vi "FORTESTING.vi"   [LabVIEW 2016, in "Test2.lvrbt"]
uses:
  Test2.lvrbt
  <vilib>/NXT/Subs/ColorSensorColors.ctl
  <vilib>/NXT/Block Support/NXT_InputPort.ctl
  <vilib>/NXT/Hardware/Plugins/Tetrix DC Motor/TetrixDCMotorAddress.ctl
  <vilib>/NXT/Hardware/Plugins/Tetrix 180 deg Servo/Tetrix180ServoAddress.ctl
  <vilib>/NXT/NXTIO Xnodes/NXTIONodeSubVIs/TETRIX IO Move DC Motors.vi
  <vilib>/NXT/Dual Mode Library/Waits/Wait_Num.vi
  <vilib>/NXT/NXTIO Xnodes/NXTIONodeSubVIs/TETRIX IO Stop DC Motors.vi
  <vilib>/NXT/Dual Mode Library/Waits/Wait_EV3_Color_Color.vi
  <vilib>/NXT/NXTIO Xnodes/NXTIONodeSubVIs/TETRIX IO Move Servos.vi
  <vilib>/NXT/Dual Mode Library/Waits/Wait_EV3_Ultrasonic_Centimeter_Closer.vi
  <vilib>/NXT/Dual Mode Library/Waits/Wait_EV3_Ultrasonic_Centimeters_Further.vi
  <vilib>/NXT/Dual Mode Library/Waits/Wait_Touch.vi
  <vilib>/NXT/Subs/LVHSConnector.ctl
  <vilib>/NXT/NXTIO Xnodes/AddressXNode/NXTIOAddress.xnode
  <vilib>/NXT/NXTIO Xnodes/NXTIOXNode/NXTIO.xnode
  <vilib>/NXT/LegoClasses/BrickReference/BrickReference.lvclass
types:
  T1 = typedef "ColorSensorColors.ctl" = enum16{"No Color", "Black", "Blue", "Green", "Yellow", "Red", "White", "Brown"}
  T2 = typedef "TetrixDCMotorAddress.ctl" = i32
  T3 = cluster{"TetrixDCMotor":T2, "TetrixDCMotor 2":T2}
  T4 = typedef "NXT_InputPort.ctl" = u32
  T5 = typedef "LVHSConnector.ctl" = refnum<class "BrickReference.lvclass">
  T6 = typedef "Tetrix180ServoAddress.ctl" = i32
  T7 = cluster{"Tetrix180Servo":T6, "Tetrix180Servo 2":T6, "Tetrix180Servo 3":T6, "Tetrix180Servo 4":T6, "Tetrix180Servo 5":T6, "Tetrix180Servo 6":T6}
  T8 = cluster{"Tetrix180Servo":T6, "Tetrix180Servo":T6, "Tetrix180Servo":T6, "Tetrix180Servo":T6, "Tetrix180Servo":T6, "Tetrix180Servo":T6}
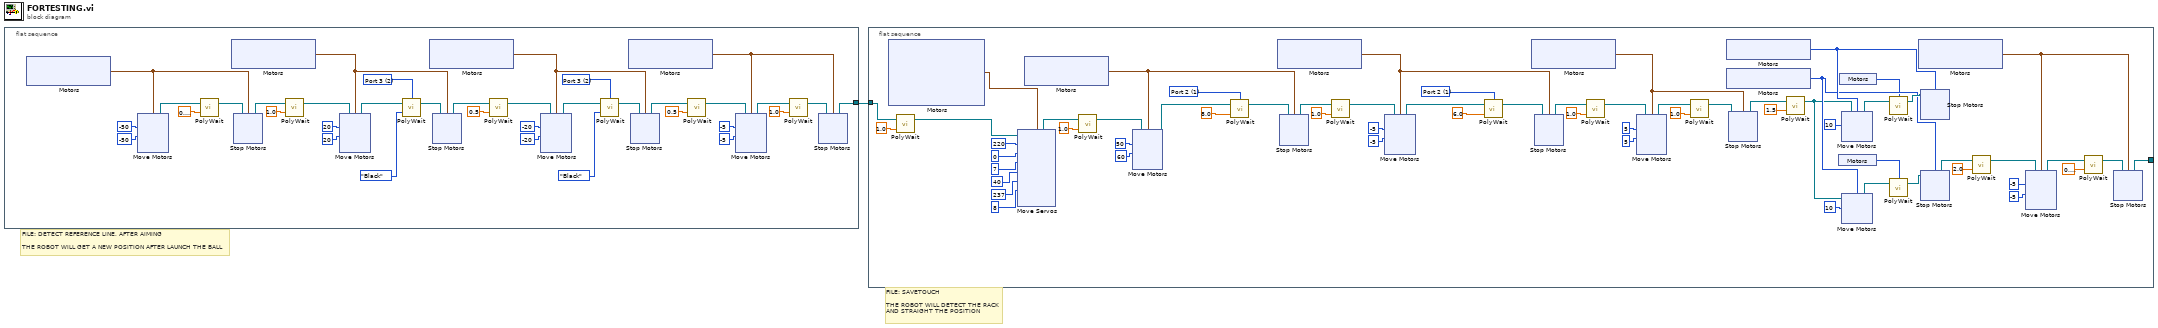
[diagram p0: block diagram]
diagram:
  # "FILE: SAVETOUCH \n\nTHE ROBOT WILL DETECT THE RACK \nAND STRAIGHT THE POSITION"
  # "FILE: DETECT REFERENCE LINE, AFTER AIMING\n\nTHE ROBOT WILL GET A NEW POSITION AFTER LAUNCH THE BALL"
  n1 = flat-sequence {
    tunnel: [w2] -> w1
    frame #0 {
      w13 = T4 2 items=["Port 1", "Port 2", "Port 3", "Port 4"] ("Port (Port 1)")
      w22 = T4 2 items=["Port 1", "Port 2", "Port 3", "Port 4"] ("Port (Port 1)")
      n2 = xnode "Motors"() -> ("Motor"=w32:cluster{"TetrixDCMotor":T2, "TetrixDCMotor":T2})
      n3 = xnode "Move Motors"("Power/Speed 2"=i8 -50, "Power/Speed 1"=i8 -50, "Motors"=w32) -> ("NXT/EV3"=w35:T5)  [unwired: 1 in]
      n4 = call-poly <vilib>:"PolyWait.vi"("Time (1 sec)"=sgl 0.8, "NXT/EV3"=w35) -> ("NXT/EV3"=w34:T5)  [unwired: 2 in]
      n5 = xnode "Motors"() -> ("Motor"=w27:cluster{"TetrixDCMotor":T2, "TetrixDCMotor":T2})
      n6 = xnode "Stop Motors"("Motors"=w32, "NXT/EV3"=w34) -> ("NXT/EV3"=w25:T5)
      n7 = call-poly <vilib>:"PolyWait.vi"("Time (1 sec)"=sgl 1.0, "NXT/EV3"=w25) -> ("NXT/EV3"=w24:T5)  [unwired: 2 in]
      n8 = xnode "Move Motors"("Power/Speed 2"=i8 20, "Power/Speed 1"=i8 20, "Motors"=w27, "NXT/EV3"=w24) -> ("NXT/EV3"=w29:T5)
      n9 = call-poly <vilib>:"PolyWait.vi"("Color (Red)"=ColorSensorColors."Black", "NXT/EV3"=w29, "Port (Port 1)"=w22) -> ("NXT/EV3"=w28:T5)  [unwired: 1 in]
      n10 = xnode "Motors"() -> ("Motor"=w17:cluster{"TetrixDCMotor":T2, "TetrixDCMotor":T2})
      n11 = xnode "Stop Motors"("Motors"=w27, "NXT/EV3"=w28) -> ("NXT/EV3"=w12:T5)
      n12 = call-poly <vilib>:"PolyWait.vi"("Time (1 sec)"=sgl 0.5, "NXT/EV3"=w12) -> ("NXT/EV3"=w15:T5)  [unwired: 2 in]
      n13 = xnode "Move Motors"("Power/Speed 2"=i8 -20, "Power/Speed 1"=i8 -20, "Motors"=w17, "NXT/EV3"=w15) -> ("NXT/EV3"=w19:T5)
      n14 = call-poly <vilib>:"PolyWait.vi"("Color (Red)"=ColorSensorColors."Black", "NXT/EV3"=w19, "Port (Port 1)"=w13) -> ("NXT/EV3"=w18:T5)  [unwired: 1 in]
      n15 = xnode "Motors"() -> ("Motor"=w6:cluster{"TetrixDCMotor":T2, "TetrixDCMotor":T2})
      n16 = xnode "Stop Motors"("Motors"=w17, "NXT/EV3"=w18) -> ("NXT/EV3"=w4:T5)
      n17 = call-poly <vilib>:"PolyWait.vi"("Time (1 sec)"=sgl 0.5, "NXT/EV3"=w4) -> ("NXT/EV3"=w3:T5)  [unwired: 2 in]
      n18 = xnode "Move Motors"("Power/Speed 2"=i8 -5, "Power/Speed 1"=i8 -5, "Motors"=w6, "NXT/EV3"=w3) -> ("NXT/EV3"=w9:T5)
      n19 = call-poly <vilib>:"PolyWait.vi"("Time (1 sec)"=sgl 1.0, "NXT/EV3"=w9) -> ("NXT/EV3"=w8:T5)  [unwired: 2 in]
      n20 = xnode "Stop Motors"("Motors"=w6, "NXT/EV3"=w8) -> ("NXT/EV3"=w2:T5)
    }
  }
  n21 = flat-sequence {
    tunnel: w1 -> [w95]
    tunnel: [w94] -> _
    frame #0 {
      w120 = T4 1 items=["Port 1", "Port 2", "Port 3", "Port 4"] ("Port (Port 1)")
      w137 = T4 1 items=["Port 1", "Port 2", "Port 3", "Port 4"] ("Port (Port 1)")
      n22 = xnode "Motors"() -> ("Motor"=w105:T8)
      n23 = call-poly <vilib>:"PolyWait.vi"("Time (1 sec)"=sgl 1.0, "NXT/EV3"=w95) -> ("NXT/EV3"=w97:T5)  [unwired: 2 in]
      n24 = xnode "Move Servos"("Position 6"=u8 8, "Position 5"=u8 237, "Position 4"=u8 40, "Position 3"=u8 7, "Position 2"=u8 0, "Position 1"=u8 220, "Motors"=w105, "NXT/EV3"=w97) -> ("NXT/EV3"=w96:T5)
      n25 = xnode "Motors"() -> ("Motor"=w150:cluster{"TetrixDCMotor":T2, "TetrixDCMotor":T2})
      n26 = call-poly <vilib>:"PolyWait.vi"("Time (1 sec)"=sgl 1.0, "NXT/EV3"=w96) -> ("NXT/EV3"=w106:T5)  [unwired: 2 in]
      n27 = xnode "Move Motors"("Power/Speed 2"=i8 60, "Power/Speed 1"=i8 50, "Motors"=w150, "NXT/EV3"=w106) -> ("NXT/EV3"=w153:T5)
      n28 = call-poly <vilib>:"PolyWait.vi"("Centimeters (40)"=sgl 8.0, "NXT/EV3"=w153, "Port (Port 1)"=w137) -> ("NXT/EV3"=w151:T5)  [unwired: 1 in]
      n29 = xnode "Motors"() -> ("Motor"=w117:cluster{"TetrixDCMotor":T2, "TetrixDCMotor":T2})
      n30 = xnode "Stop Motors"("Motors"=w150, "NXT/EV3"=w151) -> ("NXT/EV3"=w126:T5)
      n31 = call-poly <vilib>:"PolyWait.vi"("Time (1 sec)"=sgl 1.0, "NXT/EV3"=w126) -> ("NXT/EV3"=w109:T5)  [unwired: 2 in]
      n32 = xnode "Move Motors"("Power/Speed 2"=i8 -5, "Power/Speed 1"=i8 -5, "Motors"=w117, "NXT/EV3"=w109) -> ("NXT/EV3"=w123:T5)
      n33 = call-poly <vilib>:"PolyWait.vi"("Centimeters (50)"=sgl 6.0, "NXT/EV3"=w123, "Port (Port 1)"=w120) -> ("NXT/EV3"=w121:T5)  [unwired: 1 in]
      n34 = xnode "Motors"() -> ("Motor"=w111:cluster{"TetrixDCMotor":T2, "TetrixDCMotor":T2})
      n35 = xnode "Stop Motors"("Motors"=w117, "NXT/EV3"=w121) -> ("NXT/EV3"=w115:T5)
      n36 = call-poly <vilib>:"PolyWait.vi"("Time (1 sec)"=sgl 1.0, "NXT/EV3"=w115) -> ("NXT/EV3"=w114:T5)  [unwired: 2 in]
      n37 = xnode "Move Motors"("Power/Speed 2"=i8 5, "Power/Speed 1"=i8 5, "Motors"=w111, "NXT/EV3"=w114) -> ("NXT/EV3"=w113:T5)
      n38 = call-poly <vilib>:"PolyWait.vi"("Time (1 sec)"=sgl 1.0, "NXT/EV3"=w113) -> ("NXT/EV3"=w112:T5)  [unwired: 2 in]
      n39 = xnode "Motors"() -> ("Motor"=w146:T2)
      n40 = xnode "Motors"() -> ("Motor"=w142:T2)
      n41 = xnode "Stop Motors"("Motors"=w111, "NXT/EV3"=w112) -> ("NXT/EV3"=w108:T5)
      n42 = call-poly <vilib>:"PolyWait.vi"("Time (1 sec)"=sgl 1.5, "NXT/EV3"=w108) -> ("NXT/EV3"=w140:T5)  [unwired: 2 in]
      n43 = xnode "Motors"() -> ("Sensor"=w139:T4)
      n44 = xnode "Motors"() -> ("Sensor"=w138:T4)
      n45 = xnode "Move Motors"("Power/Speed 1"=i8 10, "Motors"=w146, "NXT/EV3"=w140) -> ("NXT/EV3"=w148:T5)
      n46 = xnode "Move Motors"("Power/Speed 1"=i8 10, "Motors"=w142, "NXT/EV3"=w140) -> ("NXT/EV3"=w143:T5)
      n47 = call-poly <vilib>:"PolyWait.vi"("NXT/EV3"=w148, "Port (Port 1)"=w138) -> ("NXT/EV3"=w147:T5)  [unwired: 2 in]
      n48 = call-poly <vilib>:"PolyWait.vi"("NXT/EV3"=w143, "Port (Port 1)"=w139) -> ("NXT/EV3"=w141:T5)  [unwired: 2 in]
      n49 = xnode "Motors"() -> ("Motor"=w134:cluster{"TetrixDCMotor":T2, "TetrixDCMotor":T2})
      n50 = xnode "Stop Motors"("Motors"=w146, "NXT/EV3"=w147) -> ()  [unwired: 1 out]
      n51 = xnode "Stop Motors"("Motors"=w142, "NXT/EV3"=w141) -> ("NXT/EV3"=w136:T5)
      n52 = call-poly <vilib>:"PolyWait.vi"("Time (1 sec)"=sgl 2.0, "NXT/EV3"=w136) -> ("NXT/EV3"=w132:T5)  [unwired: 2 in]
      n53 = xnode "Move Motors"("Power/Speed 2"=i8 -5, "Power/Speed 1"=i8 -5, "Motors"=w134, "NXT/EV3"=w132) -> ("NXT/EV3"=w129:T5)
      n54 = call-poly <vilib>:"PolyWait.vi"("Time (1 sec)"=sgl 0.2, "NXT/EV3"=w129) -> ("NXT/EV3"=w128:T5)  [unwired: 2 in]
      n55 = xnode "Stop Motors"("Motors"=w134, "NXT/EV3"=w128) -> ("NXT/EV3"=w94:T5)
    }
  }
